vi "ReadFGV Err.vi"(8 "error in (no error)":errorcluster, 10 "0Cv/1ST":i32, 11 "BarcodeScan in":refnum<class "BarcodeScan.lvclass">) -> (0 "error out":errorcluster, 3 "BarcodeScan out":refnum<class "BarcodeScan.lvclass">)   [LabVIEW 2019, in "BarcodeScan.lvclass"]
uses:
  BarcodeScan.lvclass
  Ctrl/Auto Inspection Data Name.ctl
  Ctrl/Auto Inspection Station Name2.ctl
  bd77d51a-16fb-4d58-85bd-3cffde9e4cef.vi
  <vilib>/JDP Science/JSONtext/JSON text to Variant.vi
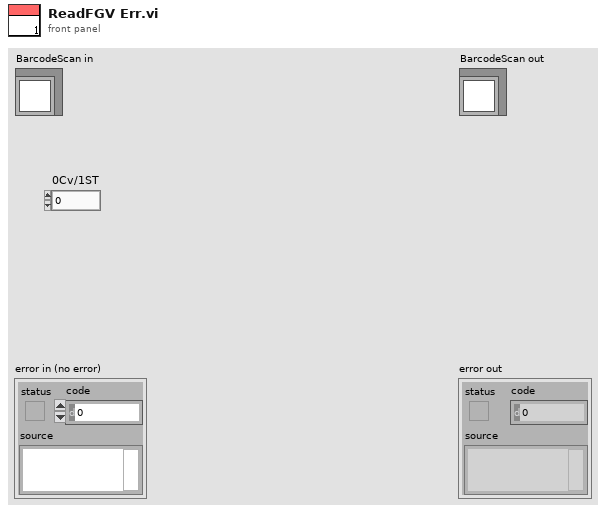
[diagram p1: front panel]
types:
  T1 = typedef "Auto Inspection Data Name.ctl" = enum16{"LocalRun", "ItemSN(TimeCode)", "CurrentAction", "Error", "Data", "OKNG", "電壓值", "電壓值判斷", "電流值", "電流值判斷", "Laser1 Data", "Laser2 Data", "Laser OKNG", "StationNO"}
  T2 = typedef "Auto Inspection Station Name2.ctl" = enum16{"S1Barcode", "S2Measure", "S3Measure", "S4Measure", "S5Measure", "S11_LaserCheck", "S8_Vision AI"}
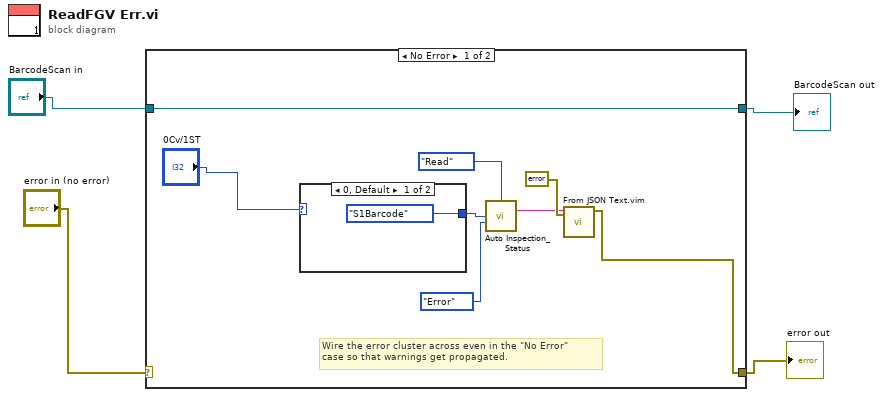
[diagram p0: block diagram]
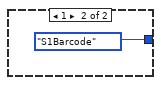
[diagram p2: hidden frame]
diagram:
  n1 = case shown="No Error" "error in (no error)" {
    selector: "error in (no error)" -> [_ w16]
    tunnel: [w6 w16] -> w1
    tunnel: [w12 w15] -> w2
    tunnel: "BarcodeScan in" -> [w12 w15]
    frame No Error {
      # "Wire the error cluster across even in the \"No Error\"\ncase so that warnings get propagated."
      n2 = case shown="0, Default" "0Cv/1ST" {
        tunnel: [Auto_Inspection_Station_Name2."S1Barcode" ("Station") Auto_Inspection_Station_Name2."S1Barcode" ("Station")] -> w8
        frame 0, Default {
        }
        frame 1 {
        }
      }
      n3 = call "Auto Inspection_Status.vi"("Action"=enum16{"Initial", "Write", "Read"}."Read", "Station"=w8, "Data"=Auto_Inspection_Data_Name."Error") -> ("DataOut"=w10:string)  [unwired: 10 in, 2 out]
      n4 = call "From JSON Text.vim"("Data Type and Default Value"=errorcluster {"status"=FALSE, "code"=0, "source"=""} ("error constant"), "JSON"=w10) -> ("Data out"=w6:errorcluster)  [unwired: 8 in, 1 out]
    }
    frame Error {
    }
  }
  "error out" <- w1
  "BarcodeScan out" <- w2
